vi "CascadedControl_src.vi"(0 "SP":T7, 1 "Gains":T5, 3 "Range":T4, 5 "PV":T6, 11 "reset":bool, 12 "ManualControl":T2) -> (4 "Vcmd":T1, 6 "Icmd":T1, 15 "Actions":T3)   [LabVIEW 2017]
uses:
  AFE/CascadeControlSetpt.ctl
  AFE/CascadeControlProcVar.ctl
  AFE/CascadeControlGains.ctl
  AFE/CascadeControlRange.ctl
  AFE/CascadeControlAction.ctl
  AFE/DQ.ctl
  AFE/ManualControl.ctl
  <vilib>/rvi/Analysis/control/PID/Typedef/niFpgaPID_PIGains.ctl
  <vilib>/rvi/Analysis/control/PID/Typedef/niFpgaPID_OutputRange.ctl
  <vilib>/rvi/Analysis/control/PID/Typedef/niFpgaPID_ManualControl.ctl
  <vilib>/rvi/Analysis/control/PID/Typedef/niFpgaPID_PIState.ctl
  <vilib>/rvi/Analysis/control/PID/Typedef/niFpgaPID_PIErrors.ctl
  AFE/ActiveFrontEnd.lvlib
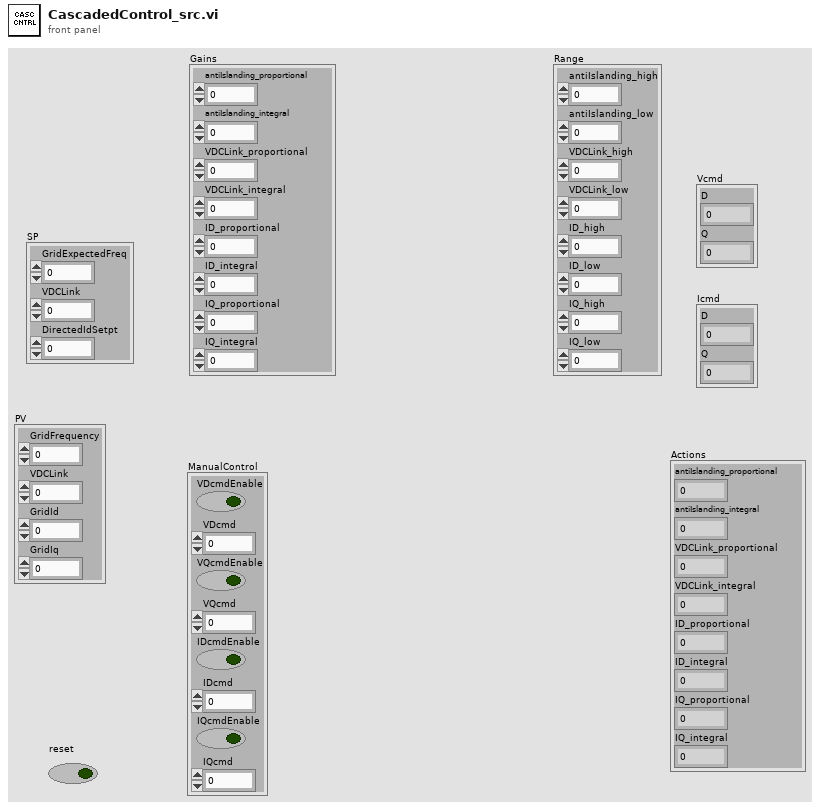
[diagram p1: front panel]
types:
  T1 = typedef "ActiveFrontEnd.lvlib/DQ.ctl" = cluster{"D":sgl, "Q":sgl}
  T2 = typedef "ActiveFrontEnd.lvlib/ManualControl.ctl" = cluster{"VDcmdEnable":bool, "VDcmd":sgl, "VQcmdEnable":bool, "VQcmd":sgl, "IDcmdEnable":bool, "IDcmd":sgl, "IQcmdEnable":bool, "IQcmd":sgl}
  T3 = typedef "ActiveFrontEnd.lvlib/CascadeControlAction.ctl" = cluster{"antiIslanding_proportional":sgl, "antiIslanding_integral":sgl, "VDCLink_proportional":sgl, "VDCLink_integral":sgl, "ID_proportional":sgl, "ID_integral":sgl, "IQ_proportional":sgl, "IQ_integral":sgl}
  T4 = typedef "ActiveFrontEnd.lvlib/CascadeControlRange.ctl" = cluster{"antiIslanding_high":sgl, "antiIslanding_low":sgl, "VDCLink_high":sgl, "VDCLink_low":sgl, "ID_high":sgl, "ID_low":sgl, "IQ_high":sgl, "IQ_low":sgl}
  T5 = typedef "ActiveFrontEnd.lvlib/CascadeControlGains.ctl" = cluster{"antiIslanding_proportional":sgl, "antiIslanding_integral":sgl, "VDCLink_proportional":sgl, "VDCLink_integral":sgl, "ID_proportional":sgl, "ID_integral":sgl, "IQ_proportional":sgl, "IQ_integral":sgl}
  T6 = typedef "ActiveFrontEnd.lvlib/CascadeControlProcVar.ctl" = cluster{"GridFrequency":sgl, "VDCLink":sgl, "GridId":sgl, "GridIq":sgl}
  T7 = typedef "ActiveFrontEnd.lvlib/CascadeControlSetpt.ctl" = cluster{"GridExpectedFreq":sgl, "VDCLink":sgl, "DirectedIdSetpt":sgl}
  T8 = typedef "niFpgaPID_PIState.ctl" = cluster{"uI(k-1)":sgl, "e(k-1)":sgl, "output (k-1)":sgl}
  T9 = typedef "niFpgaPID_ManualControl.ctl" = cluster{"manual? (F)":bool, "manual input (0)":sgl}
  T10 = typedef "niFpgaPID_OutputRange.ctl" = cluster{"output high (Inf)":sgl, "output low (-Inf)":sgl}
  T11 = typedef "niFpgaPID_PIGains.ctl" = cluster{"proportional gain":sgl, "integral gain":sgl}
  T12 = typedef "niFpgaPID_PIErrors.ctl" = cluster{"error":sgl, "error with beta":sgl}
  T13 = typedef "niFpgaPID_PIActions.ctl" = cluster{"proportional action":sgl, "integral action":sgl}
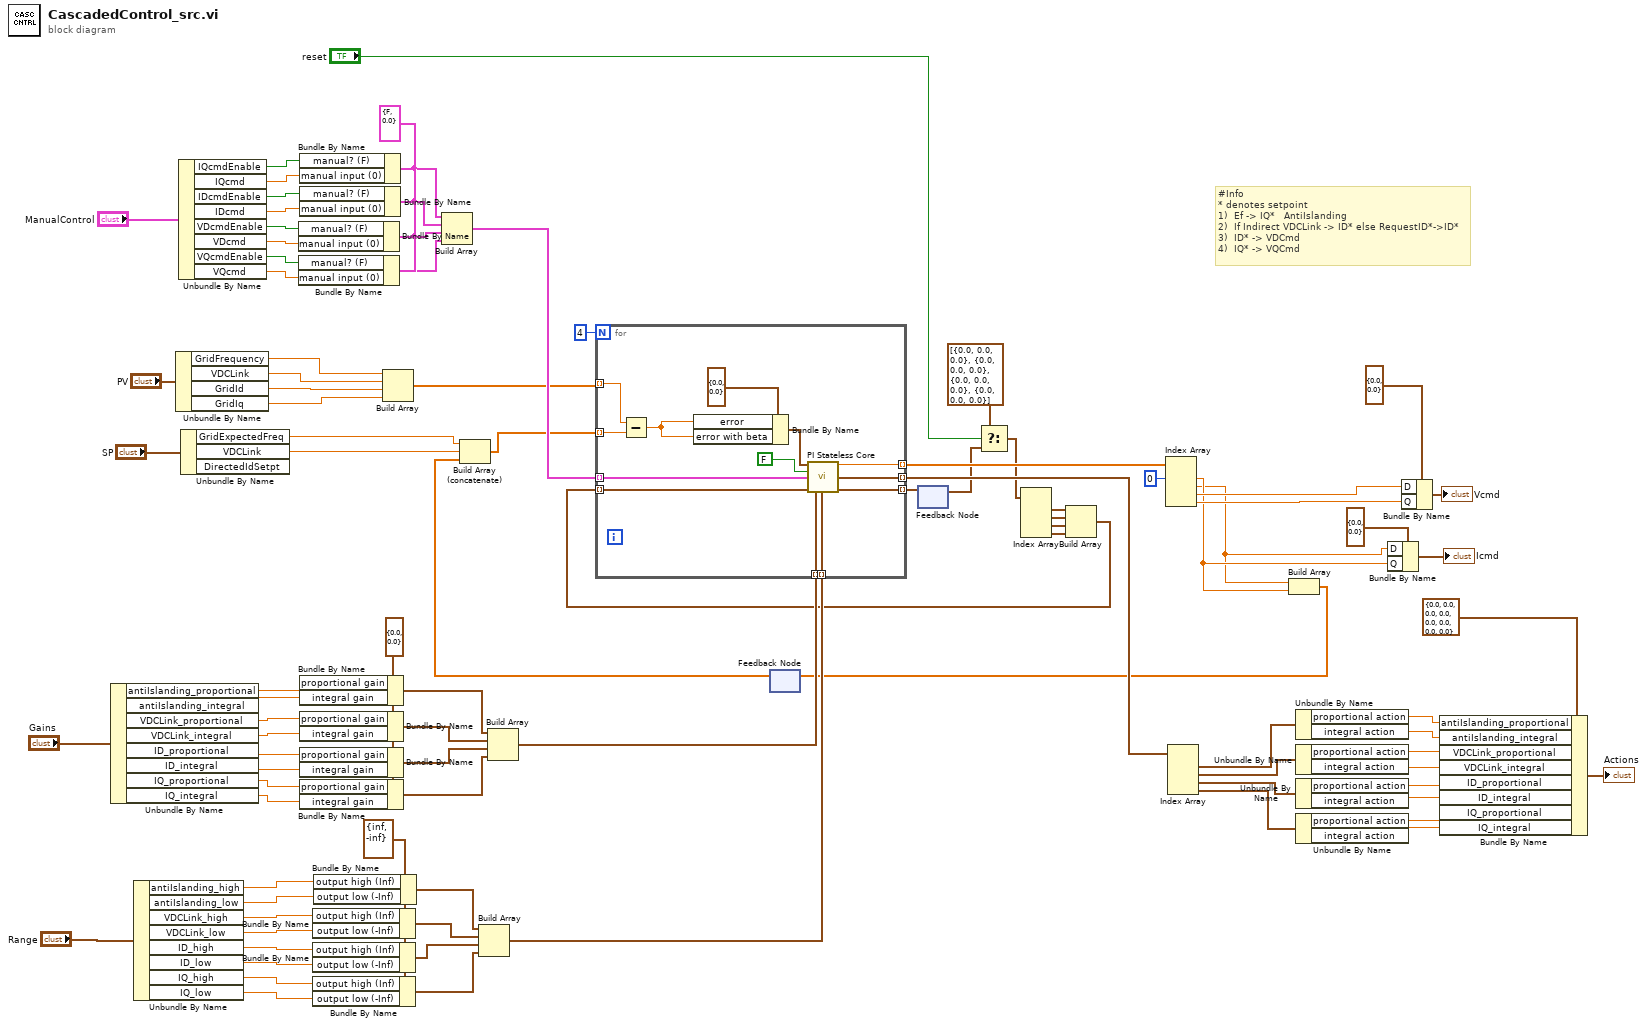
[diagram p0: block diagram]
diagram:
  w36 = T9 {"manual? (F)"=FALSE, "manual input (0)"=0.0} ("manual control")
  w71 = T10 {"output high (Inf)"=inf, "output low (-Inf)"=-inf} ("output range")
  w81 = T11 {"proportional gain"=0.0, "integral gain"=0.0} ("gains")
  # "#Info\n* denotes setpoint\n1)  Ef -> IQ*   AntiIslanding\n2)  If Indirect VDCLink -> ID* else RequestID*->ID*\n3)  ID* -> VDCmd\n4)  IQ* -> VQCmd"
  n1 = Unbundle By Name("Gains") -> ("antiIslanding_proportional"=w85:sgl, "antiIslanding_integral"=w84:sgl, "VDCLink_proportional"=w83:sgl, "VDCLink_integral"=w82:sgl, "ID_proportional"=w78:sgl, "ID_integral"=w77:sgl, "IQ_proportional"=w80:sgl, "IQ_integral"=w79:sgl)
  n2 = Unbundle By Name("Range") -> ("antiIslanding_high"=w69:sgl, "antiIslanding_low"=w68:sgl, "VDCLink_high"=w67:sgl, "VDCLink_low"=w66:sgl, "ID_high"=w65:sgl, "ID_low"=w64:sgl, "IQ_high"=w63:sgl, "IQ_low"=w62:sgl)
  n3 = Unbundle By Name("PV") -> ("GridFrequency"=w37:sgl, "VDCLink"=w92:sgl, "GridId"=w91:sgl, "GridIq"=w90:sgl)
  n4 = Unbundle By Name("ManualControl") -> ("IQcmdEnable"=w30:bool, "IQcmd"=w29:sgl, "IDcmdEnable"=w28:bool, "IDcmd"=w27:sgl, "VDcmdEnable"=w26:bool, "VDcmd"=w25:sgl, "VQcmdEnable"=w24:bool, "VQcmd"=w23:sgl)
  n5 = Unbundle By Name("SP") -> ("GridExpectedFreq"=w21:sgl, "VDCLink"=w20:sgl)  [unwired: 1 out]
  n6 = Bundle By Name(cluster=w36, "manual? (F)"=w26, "manual input (0)"=w25) -> (w33:T9)
  n7 = Bundle By Name(cluster=w36, "manual? (F)"=w24, "manual input (0)"=w23) -> (w32:T9)
  n8 = Bundle By Name(cluster=w36, "manual? (F)"=w30, "manual input (0)"=w29) -> (w35:T9)
  n9 = Bundle By Name(cluster=w36, "manual? (F)"=w28, "manual input (0)"=w27) -> (w34:T9)
  n10 = Bundle By Name(cluster=w81, "proportional gain"=w85, "integral gain"=w84) -> (w76:T11)
  n11 = Bundle By Name(cluster=w81, "proportional gain"=w83, "integral gain"=w82) -> (w75:T11)
  n12 = Bundle By Name(cluster=w81, "proportional gain"=w78, "integral gain"=w77) -> (w74:T11)
  n13 = Bundle By Name(cluster=w81, "proportional gain"=w80, "integral gain"=w79) -> (w73:T11)
  n14 = Bundle By Name(cluster=w71, "output high (Inf)"=w67, "output low (-Inf)"=w66) -> (w60:T10)
  n15 = Bundle By Name(cluster=w71, "output high (Inf)"=w65, "output low (-Inf)"=w64) -> (w59:T10)
  n16 = Bundle By Name(cluster=w71, "output high (Inf)"=w63, "output low (-Inf)"=w62) -> (w58:T10)
  n17 = Bundle By Name(cluster=w71, "output high (Inf)"=w69, "output low (-Inf)"=w68) -> (w61:T10)
  n18 = Build Array(w37, w92, w91, w90) -> (w7:sgl[])
  n19 = Build Array(w35, w34, w33, w32) -> (w22:T9[])
  n20 = Build Array(w61, w60, w59, w58) -> (w57:T10[])
  n21 = Build Array(w76, w75, w74, w73) -> (w72:T11[])
  n22 = feedback #1() -> (w19:sgl[])  [unwired: 1 in]
  n23 = Build Array (concatenate)(w21, w20, w19) -> (w6:sgl[])
  n24 = feedback #2() -> (w11:T8[])  [unwired: 1 in]
  n25 = Select(t=T8[] [{"uI(k-1)"=0.0, "e(k-1)"=0.0, "output (k-1)"=0.0}, {"uI(k-1)"=0.0, "e(k-1)"=0.0, "output (k-1)"=0.0}, {"uI(k-1)"=0.0, "e(k-1)"=0.0, "output (k-1)"=0.0}, {"uI(k-1)"=0.0, "e(k-1)"=0.0, "output (k-1)"=0.0}], s="reset", f=w11) -> (s? t:f=w8:T8[])
  n26 = Index Array(array=w8) -> (element #1=w16:T8, element #2=w15:T8, element #3=w14:T8, element #4=w13:T8)  [unwired: 4 in]
  n27 = Build Array(w16, w15, w14, w13) -> (w12:T8[])
  n28 = for {
    N: 4 -> [_]
    tunnel: w12 -> [w97] mode=indexing
    tunnel: [w96] -> w88 mode=indexing
    tunnel: w72 -> [w100] mode=indexing
    tunnel: w57 -> [w99] mode=indexing
    tunnel: [w95] -> w56 mode=indexing
    tunnel: w7 -> [w105] mode=indexing
    tunnel: w6 -> [w104] mode=indexing
    tunnel: w22 -> [w98] mode=indexing
    tunnel: [w94] -> w17 mode=indexing
    n29 = Subtract(x=w105, y=w104) -> (x-y=w103:sgl)
    n30 = Bundle By Name(cluster=T12 {"error"=0.0, "error with beta"=0.0} ("errors"), "error"=w103, "error with beta"=w103) -> (w102:T12)
    n31 = call "PI Stateless Core"("errors"=w102, "enable bumpless transfer? (F)"=FALSE, "manual control"=w98, "state in"=w97, "gains"=w100, "output range"=w99) -> ("output"=w96:sgl, "actions"=w95:T13, "state out"=w94:T8)  [unwired: 6 in, 1 out]
  }
  n32 = feedback-in #2(w17) -> ()
  n33 = Index Array(array=w88, index #1=0 ("index")) -> (element #1=w3:sgl, element #2=w2:sgl, element #3=w39:sgl, element #4=w38:sgl)  [unwired: 3 in]
  n34 = Index Array(array=w56) -> (element #1=w55:T13, element #2=w54:T13, element #3=w53:T13, element #4=w52:T13)  [unwired: 4 in]
  n35 = Build Array(w2, w3) -> (w4:sgl[])
  n36 = feedback-in #1(w4) -> ()
  n37 = Unbundle By Name(w55) -> ("proportional action"=w50:sgl, "integral action"=w49:sgl)
  n38 = Unbundle By Name(w54) -> ("proportional action"=w48:sgl, "integral action"=w47:sgl)
  n39 = Unbundle By Name(w53) -> ("proportional action"=w46:sgl, "integral action"=w45:sgl)
  n40 = Unbundle By Name(w52) -> ("proportional action"=w44:sgl, "integral action"=w43:sgl)
  n41 = Bundle By Name(cluster=T1 {"D"=0.0, "Q"=0.0} ("DQ"), "D"=w2, "Q"=w3) -> (→"Icmd":T1)
  n42 = Bundle By Name(cluster=T1 {"D"=0.0, "Q"=0.0} ("DQ"), "D"=w39, "Q"=w38) -> (→"Vcmd":T1)
  n43 = Bundle By Name(cluster=T3 {"antiIslanding_proportional"=0.0, "antiIslanding_integral"=0.0, "VDCLink_proportional"=0.0, "VDCLink_integral"=0.0, "ID_proportional"=0.0, "ID_integral"=0.0, "IQ_proportional"=0.0, "IQ_integral"=0.0} ("Action"), "antiIslanding_proportional"=w50, "antiIslanding_integral"=w49, "VDCLink_proportional"=w48, "VDCLink_integral"=w47, "ID_proportional"=w46, "ID_integral"=w45, "IQ_proportional"=w44, "IQ_integral"=w43) -> (→"Actions":T3)
